vi "sub vi dzailajace.vi"(11 "Enum in":T1) -> (3 "Array 2":dbl[][](array[numeric]))   [LabVIEW 2020]
uses:
  Control 4.ctl
  <vilib>/Utility/file.llb/Write Delimited Spreadsheet (DBL).vi
  <vilib>/Utility/file.llb/Read Delimited Spreadsheet (DBL).vi
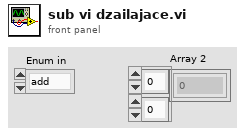
[diagram p1: front panel]
types:
  T1 = typedef "Control 4.ctl" = enum16{"add", "read", "readAll", "reset", "zapis_do_pliku", "odczyt_z_pliku"}
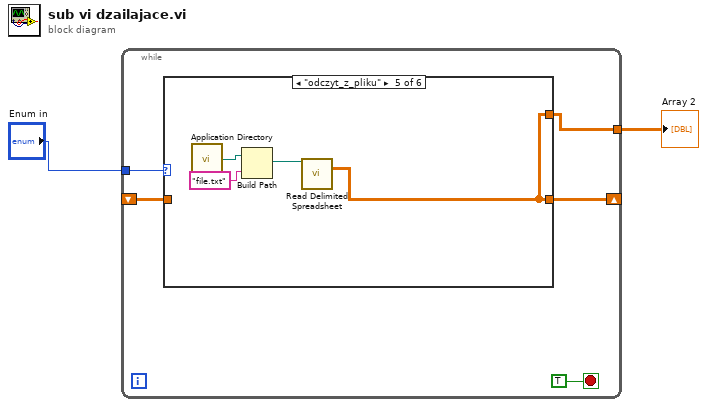
[diagram p0: block diagram]
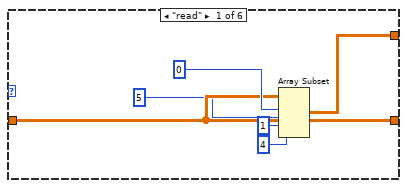
[diagram p2: hidden frame]
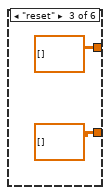
[diagram p4: hidden frame]
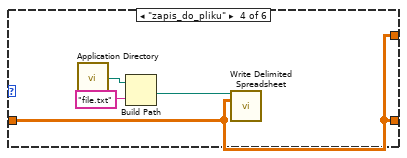
[diagram p5: hidden frame]
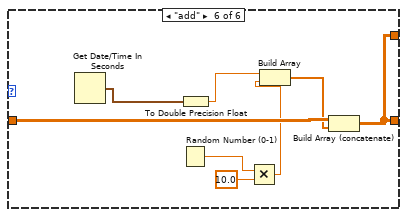
[diagram p6: hidden frame]
diagram:
  n1 = while {
    tunnel: "Enum in" -> [w6]
    shift-right: [w4] -> _
    shift-left: _ -> [w5]
    tunnel: [w3] -> w2
    stop <- TRUE stop-if-true
    n2 = case shown="\"odczyt_z_pliku\"" w6 {
      tunnel: w5 -> [w12 w14 _ w20 _ w30]
      tunnel: [w12 w14 dbl[][] [] w20 w24 w28] -> w4
      tunnel: [w11 w14 dbl[][] [] w20 w24 w28] -> w3
      frame "read" {
        n3 = Array Subset(array=w12, index (row)=0 ("index"), length (row)=5 ("length"), index (col)=1 ("index"), length (col)=4 ("length")) -> (w11:dbl[][])
      }
      frame "readAll" {
      }
      frame "reset" {
      }
      frame "zapis_do_pliku" {
        n4 = call <vilib>:"Application Directory.vi"() -> ("Application Directory"=w19:path)
        n5 = Build Path(base path=w19, name or relative path="file.txt") -> (appended path=w17:path)
        n6 = call-poly <vilib>:"Write Delimited Spreadsheet.vi"("file path (dialog if empty)"=w17, "2D data"=w20) -> ()  [unwired: 12 in, 2 out]
      }
      frame "odczyt_z_pliku" {
        n7 = call <vilib>:"Application Directory.vi"() -> ("Application Directory"=w22:path)
        n8 = Build Path(base path=w22, name or relative path="file.txt") -> (appended path=w23:path)
        n9 = call-poly <vilib>:"Read Delimited Spreadsheet.vi"("file path (dialog if empty)"=w23) -> ("all rows"=w24:dbl[][])  [unwired: 9 in, 5 out]
      }
      frame "add" {
        n10 = Get Date/Time In Seconds() -> (seconds since 1Jan1904=w32:timestamp)
        n11 = Random Number (0-1)() -> (number: 0 to 1=w25:dbl)
        n12 = To Double Precision Float(number=w32) -> (double precision float=w31:dbl)
        n13 = Multiply(x=w25, y=10.0) -> (x*y=w26:dbl)
        n14 = Build Array(w31, w26) -> (w29:dbl[])
        n15 = Build Array (concatenate)(w30, w29) -> (w28:dbl[][])
      }
    }
  }
  "Array 2" <- w2
